vi "Graph_TraceSelect_CheckBox.vi"(10 "Checkbox Cluster":T1={"Boolean"=TRUE, "Boolean 2"=TRUE, "Boolean 3"=TRUE, "Boolean 4"=TRUE, "Boolean 5"=FALSE, "Boolean 6"=FALSE, "Boolean 7"=FALSE, "Boolean 8"=FALSE}, 11 "Input Signals":waveform(dbl)[](array[waveform])) -> (3 "Array":waveform(dbl)[](array[waveform]))   [LabVIEW 2013]
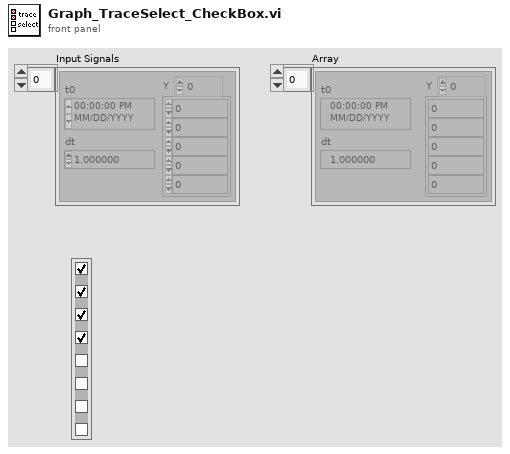
[diagram p1: front panel]
types:
  T1 = cluster{"Boolean":bool, "Boolean 2":bool, "Boolean 3":bool, "Boolean 4":bool, "Boolean 5":bool, "Boolean 6":bool, "Boolean 7":bool, "Boolean 8":bool}
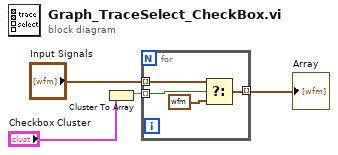
[diagram p0: block diagram]
diagram:
  n1 = Cluster To Array(cluster="Checkbox Cluster") -> (array=w3:bool[])
  n2 = for {
    tunnel: "Input Signals" -> [w8] mode=indexing
    tunnel: w3 -> [w6] mode=indexing
    tunnel: [w5] -> w4 mode=indexing
    n3 = Select(t=w8, s=w6, f=waveform(dbl) {"t0"=timestamp(0 s since 1904-01-01), "dt"=1.0, "Y"=[]}) -> (s? t:f=w5:waveform(dbl))
  }
  "Array" <- w4
